vi "Puff_using_Arduino.vi"() -> (5 "Plug in titles":string[](array[string]), 7 "Plug in values":string[](array[string]))   [LabVIEW 2014]
uses:
  Globals/Meas_global.vi
panel:
  # "By selecting this vi to run you are telling Data Translation.vi to use the Puff with Arduino vi."
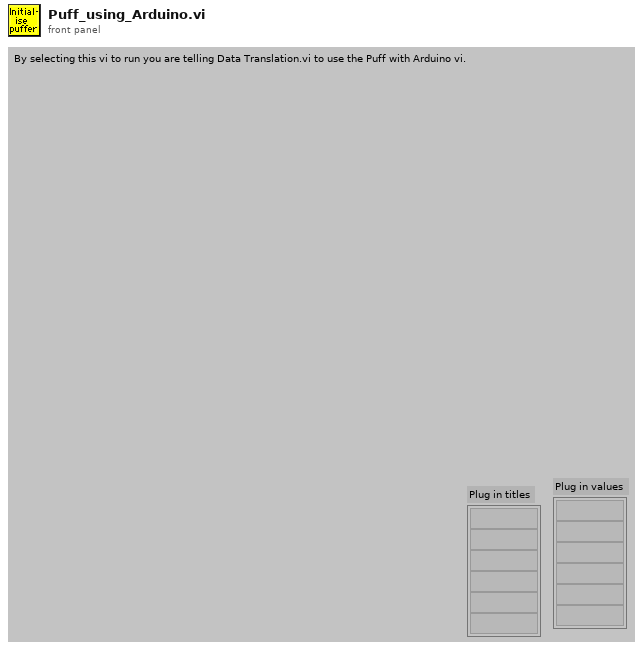
[diagram p1: front panel]
types:
  T1 = typedef "Post_Process.ctl" = enum16{"Take New Data", "Post Process Raw Data File"}
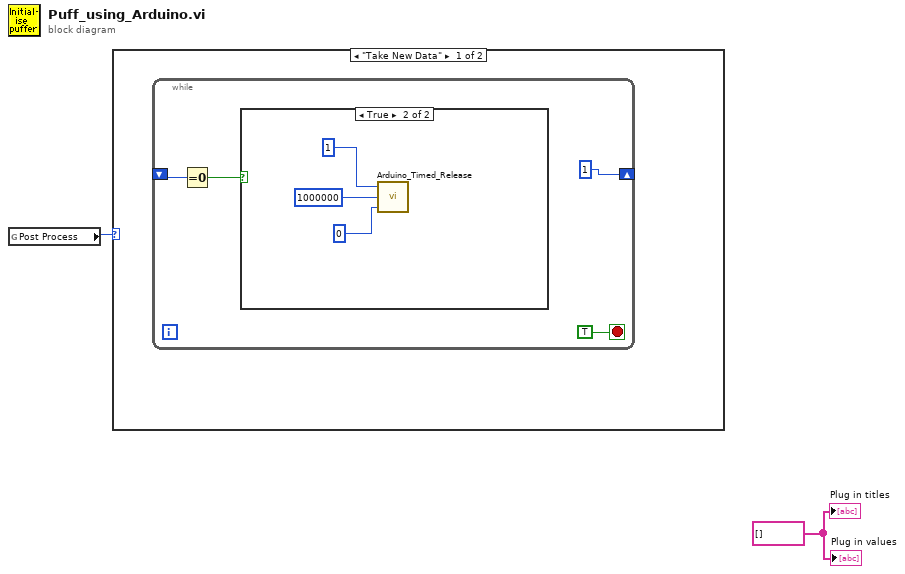
[diagram p0: block diagram]
diagram:
  w2 = string[] [] ("Plug in titles")
  n1 = global read "Meas_global.vi" "Post Process"() -> (w1:T1)
  n2 = case shown="\"Take New Data\"" w1 {
    frame "Take New Data" {
      n3 = while {
        shift-right: [1] -> _
        shift-left: _ -> [w5]
        stop <- TRUE stop-if-true
        n4 = Equal To 0?(x=w5) -> (x = 0?=w4:bool)
        n5 = case shown="True" w4 {
          frame False {
          }
          frame True {
            n6 = call "Arduino_Timed_Release.vi"("Time to hold source ON (microseconds)"=u32 0 ("Time to hold source OFF (microseconds)"), "Time to hold source OFF (microseconds)"=u32 1000000, "Number of cycles"=u16 1) -> ()  [unwired: 2 out]
          }
        }
      }
    }
    frame "Post Process Raw Data File" {
    }
  }
  "Plug in values" <- w2
  "Plug in titles" <- w2
